vi "fgt get sensor Range.vi"(8 "error in (no error)":errorcluster, 11 "sensorIndex":u32) -> (0 "error out":errorcluster, 2 "Smax out":sgl, 3 "Smin out":sgl)   [LabVIEW 2020, in "fgt_SDK.lvlib"]
doc: "Get sensor minimum and maximum range. Returned values takes into account set unit, default value is 'µl/min' in case of flow-units and 'mbar' for pressure sensors."
uses:
  fgt_SDK.lvlib
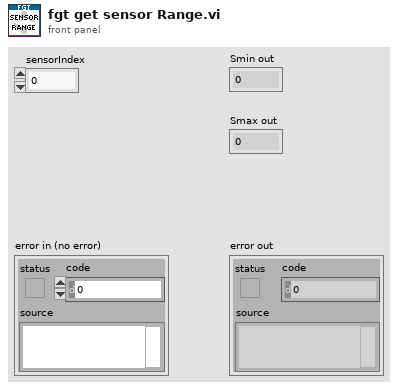
[diagram p1: front panel]
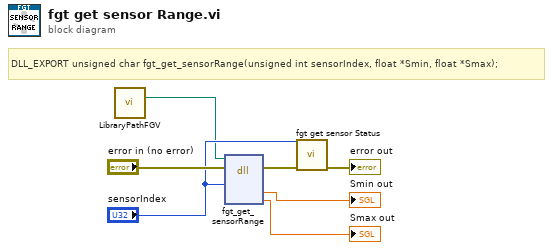
[diagram p0: block diagram]
diagram:
  # "DLL_EXPORT unsigned char fgt_get_sensorRange(unsigned int sensorIndex, float *Smin, float *Smax);"
  n1 = call "LibraryPathFGV.vi"() -> ("Path Out"=w1:path)  [unwired: 14 in, 1 out]
  n2 = dll-call lib="C:/Workspace/fgt-SDK/LabVIEW/dlls/fgt_SDK_*.*" fn="fgt_get_sensorRange"(path in=w1, error in="error in (no error)", "sensorIndex"="sensorIndex") -> (error out=w4:errorcluster, "Smin"=→"Smin out":sgl, "Smax"=→"Smax out":sgl)  [unwired: 5 in, 1 out]
  n3 = call "fgt get sensor Status.vi"("error in (no error)"=w4, "pressureIndex"="sensorIndex") -> ("error out"=→"error out":errorcluster)  [unwired: 9 in]
